vi "Runtime Parameters.vi"() -> ()   [LabVIEW 2020]
uses:
  Runtime Parameters.ctl
panel:
  in  "Runtime Parameters":T1={"Scale Bar"=TRUE, "ScaleBarSize"=10.0, "XYIncreatement+"=40.0, "ZIncreatement++"=5.0, "Autostretch"=FALSE, "Binning"=0.0, "ZIncreatement+"=0.2, "MicroStage+"=100.0, "Exposure"=200.0, "Interval"=200.0, "XYIncreatement++"=80.0, "CaptureFrame"=500.0} {"CaptureFrame" format="%#_13g"; "XYIncreatement++" format="%#_13g"; "Interval" format="%#_13g"; "Exposure" format="%#_13g"; "MicroStage+" format="%#_13g"; "ZIncreatement+" format="%#_13g"; "Binning" format="%#_13g"; "ZIncreatement++" format="%#_13g"; "XYIncreatement+" format="%#_13g"; "ScaleBarSize" format="%#_13g"}
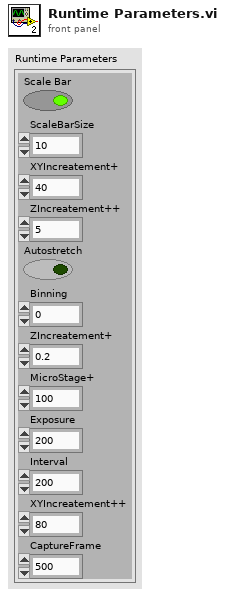
[diagram p1: front panel]
types:
  T1 = typedef "Runtime Parameters.ctl" = cluster{"Scale Bar":bool, "ScaleBarSize":dbl, "XYIncreatement+":dbl, "ZIncreatement++":dbl, "Autostretch":bool, "Binning":dbl, "ZIncreatement+":dbl, "MicroStage+":dbl, "Exposure":dbl, "Interval":dbl, "XYIncreatement++":dbl, "CaptureFrame":dbl}
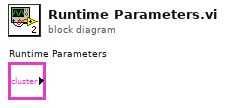
[diagram p0: block diagram]
diagram:
